vi "ReadSizeNchwMat_U8.vi"(8 "error in":errorcluster, 11 "Array":u8[][][][](array[numeric])) -> (0 "error out":errorcluster, 1 "Channels":i32, 2 "Dimensions":i32, 3 "Array":u8[][][][](array[numeric]), 4 "Height":i32, 6 "Width":i32)   [LabVIEW 2020, in "OpenLvVision_OpenCv.lvlib"]
uses:
  OpenLvVision_OpenCv.lvlib
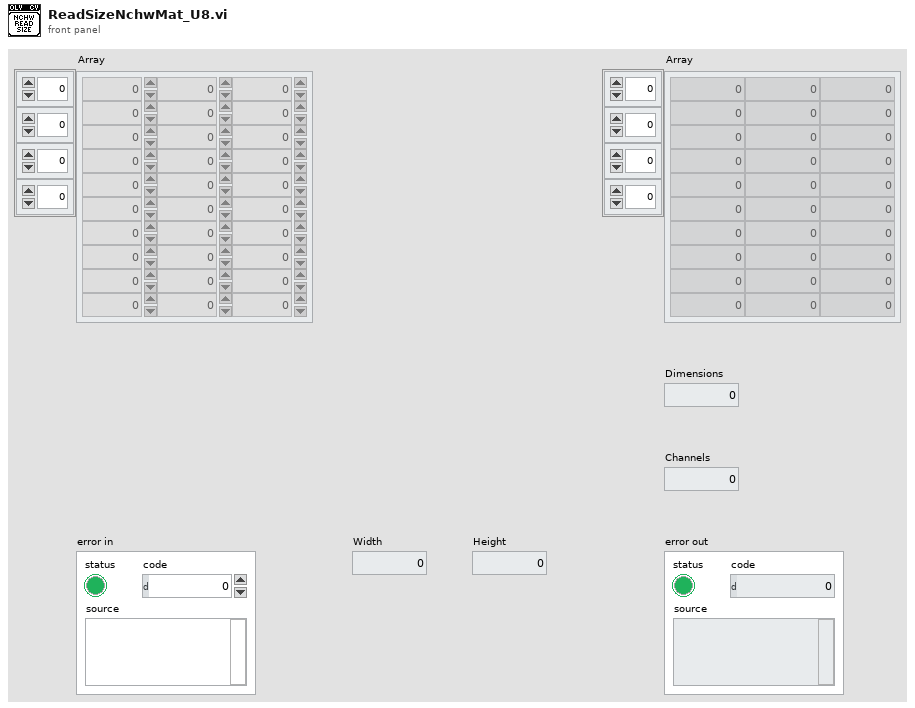
[diagram p1: front panel]
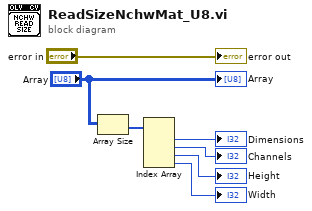
[diagram p0: block diagram]
diagram:
  n1 = Array Size(array="Array") -> (size(s)=w5:i32[])
  n2 = Index Array(array=w5) -> (element #1=→"Dimensions":i32, element #2=→"Channels":i32, element #3=→"Height":i32, element #4=→"Width":i32)  [unwired: 4 in]
  "Array" <- "Array"
  "error out" <- "error in"
